vi "Main.vi"   [LabVIEW 2018, in "Temp Recipe.lvlib" / "Recipe Editor.lvclass"]
uses:
  Recipe Editor.lvclass
panel:
  # "Editor Main"
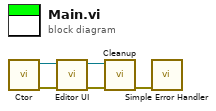
[diagram p0: block diagram]
diagram:
  n1 = call "Ctor.vi"() -> ("error out"=w4:errorcluster, "Class"=w5:refnum<class "Recipe Editor.lvclass">)  [unwired: 10 in]
  n2 = call "Editor UI.vi"("error in (no error)"=w4, "Recipe Editor in"=w5) -> ("error out"=w2:errorcluster, "Recipe Editor out"=w3:refnum<class "Recipe Editor.lvclass">)  [unwired: 8 in]
  n3 = call "Cleanup.vi"("error in (no error)"=w2, "Class In"=w3) -> ("error out"=w1:errorcluster)  [unwired: 9 in]
  n4 = call <vilib>:"Simple Error Handler.vi"("error in (no error)"=w1) -> ()  [unwired: 4 in, 5 out]
